vi "Score and Rank Target Objects.vi"(8 "Annotate":bool, 9 "Score Limit":dbl=70.0, 10 "Particles":T4(array[cluster]), 11 "Image in":T3) -> (0 "Target Info":T2(array[cluster]), 3 "Annotated Image":T3)   [LabVIEW 2013]
doc: "Use the location, size, and other factors to score and rank the objects. Optionally show annotations over the objects."
uses:
  <vilib>/vision/Image Controls.llb/IMAQ Image.ctl
  TargetType.ctl
panel:
  out "Numeric":i32
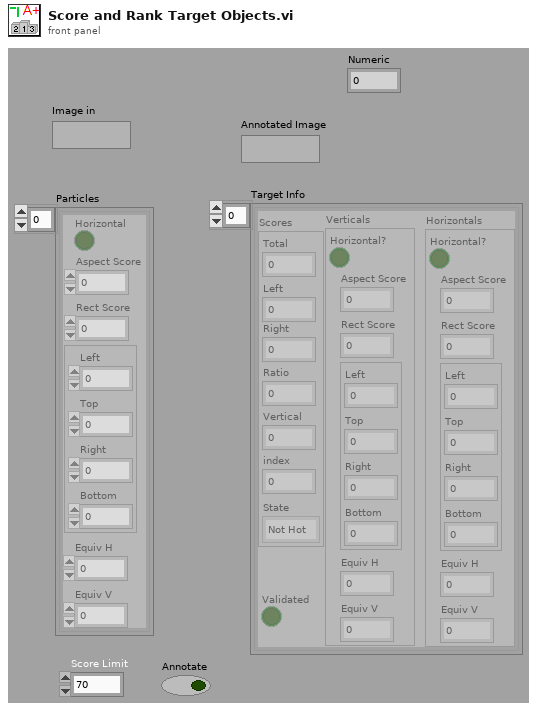
[diagram p1: front panel]
types:
  T1 = typedef "TargetType.ctl" = enum16{"Not Hot", "Hot"}
  T2 = cluster{"Scores":cluster{"Total":dbl, "Left":dbl, "Right":dbl, "Ratio":dbl, "Vertical":dbl, "index":i32, "State":T1}, "Verticals":cluster{"Horizontal?":bool, "Aspect Score":dbl, "Rect Score":dbl, cluster{"Left":dbl, "Top":dbl, "Right":dbl, "Bottom":dbl}, "Equiv H":dbl, "Equiv V":dbl}, "Horizontals":cluster{"Horizontal?":bool, "Aspect Score":dbl, "Rect Score":dbl, cluster{"Left":dbl, "Top":dbl, "Right":dbl, "Bottom":dbl}, "Equiv H":dbl, "Equiv V":dbl}, "Validated":bool}[]
  T3 = typedef "IMAQ Image.ctl" = refnum<image>
  T4 = cluster{"Horizontal":bool, "Aspect Score":dbl, "Rect Score":dbl, cluster{"Left":dbl, "Top":dbl, "Right":dbl, "Bottom":dbl}, "Equiv H":dbl, "Equiv V":dbl}[]
  T5 = cluster{cluster{dbl, dbl, dbl, dbl, dbl, i32, T1}, cluster{"Horizontal":bool, "Aspect Score":dbl, "Rect Score":dbl, cluster{"Left":dbl, "Top":dbl, "Right":dbl, "Bottom":dbl}, "Equiv H":dbl, "Equiv V":dbl}, cluster{"Horizontal":bool, "Aspect Score":dbl, "Rect Score":dbl, cluster{"Left":dbl, "Top":dbl, "Right":dbl, "Bottom":dbl}, "Equiv H":dbl, "Equiv V":dbl}, bool}[]
  T6 = cluster{"Score":dbl, cluster{"Horizontal":bool, "Aspect Score":dbl, "Rect Score":dbl, cluster{"Left":dbl, "Top":dbl, "Right":dbl, "Bottom":dbl}, "Equiv H":dbl, "Equiv V":dbl}}[]
  T7 = cluster{"Horizontal":bool, "Aspect Score":dbl, "Rect Score":dbl, cluster{"Left":dbl, "Top":dbl, "Right":dbl, "Bottom":dbl}, "Equiv H":dbl, "Equiv V":dbl}
  T8 = cluster{cluster{dbl, dbl, dbl, dbl, dbl, i32, T1}, cluster{"Horizontal":bool, "Aspect Score":dbl, "Rect Score":dbl, cluster{"Left":dbl, "Top":dbl, "Right":dbl, "Bottom":dbl}, "Equiv H":dbl, "Equiv V":dbl}, cluster{"Horizontal":bool, "Aspect Score":dbl, "Rect Score":dbl, cluster{"Left":dbl, "Top":dbl, "Right":dbl, "Bottom":dbl}, "Equiv H":dbl, "Equiv V":dbl}, bool}
  T9 = cluster{"Score":dbl, cluster{"Horizontal":bool, "Aspect Score":dbl, "Rect Score":dbl, cluster{"Left":dbl, "Top":dbl, "Right":dbl, "Bottom":dbl}, "Equiv H":dbl, "Equiv V":dbl}}
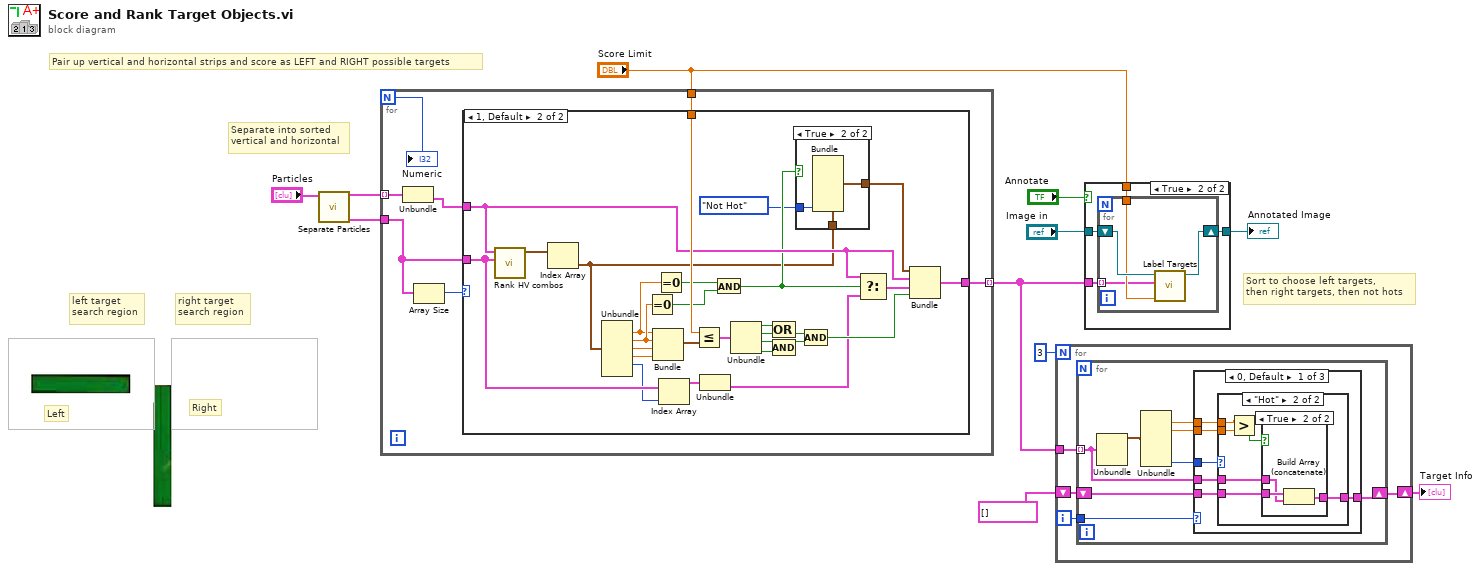
[diagram p0: block diagram]
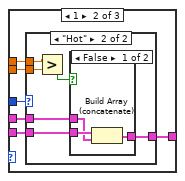
[diagram p5: hidden frame]
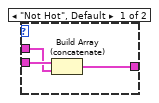
[diagram p9: hidden frame]
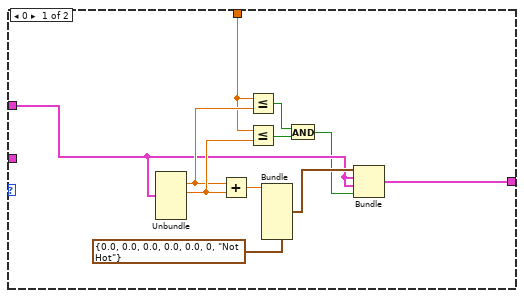
[diagram p10: hidden frame]
diagram:
  # "Sort to choose left targets,\nthen right targets, then not hots"
  # "Right"
  # "Left"
  # "right target\nsearch region"
  # "left target\nsearch region"
  # "Separate into sorted\nvertical and horizontal"
  # "Pair up vertical and horizontal strips and score as LEFT and RIGHT possible targets"
  n1 = call "Separate Particles.vi"("Objects"="Particles") -> ("H Scores"=w7:T6, "V Scores"=w8:T6)  [unwired: 9 in]
  n2 = for {
    N -> [w12]
    tunnel: w8 -> [w18] mode=indexing
    tunnel: w7 -> [w16]
    tunnel: [w14] -> w5 mode=indexing
    tunnel: "Score Limit" -> [w13]
    n3 = Unbundle(w18) -> (w17:T7)  [unwired: 1 out]
    n4 = Array Size(array=w16) -> (size(s)=w15:i32)
    n5 = case shown="1, Default" w15 {
      tunnel: w16 -> [_ w44]
      tunnel: w17 -> [w23 w34]
      tunnel: [w21 w42] -> w14
      tunnel: w13 -> [w20 w41]
      frame 0 {
        n6 = Unbundle(w23) -> ("Aspect Score"=w26:dbl, "Rect Score"=w27:dbl)  [unwired: 4 out]
        n7 = Add(x=w26, y=w27) -> (x+y=w25:dbl)
        n8 = Less Or Equal?(x=w20, y=w26) -> (x <= y?=w28:bool)
        n9 = Less Or Equal?(x=w20, y=w27) -> (x <= y?=w29:bool)
        n10 = Bundle(cluster=cluster{dbl, dbl, dbl, dbl, dbl, i32, T1} {0.0, 0.0, 0.0, 0.0, 0.0, 0, enum."Not Hot"}, w25) -> (w24:cluster{dbl, dbl, dbl, dbl, dbl, i32, T1})  [unwired: 6 in]
        n11 = And(x=w28, y=w29) -> (x .and. y?=w22:bool)
        n12 = Bundle(w24, w23, w23, w22) -> (w21:T8)  [unwired: 1 in]
      }
      frame 1, Default {
        n13 = call "Rank HV combos.vi"("H Scores"=w44, "Vertical"=w34) -> ("Target Scores"=w57:cluster{dbl, dbl, dbl, dbl, dbl, i32, T1}[])  [unwired: 9 in]
        n14 = Index Array(array=w57) -> (element=w30:cluster{dbl, dbl, dbl, dbl, dbl, i32, T1})  [unwired: 1 in]
        n15 = Unbundle(w30) -> (w39:dbl, w40:dbl, w53:dbl, w54:dbl, w43:i32)  [unwired: 2 out]
        n16 = Equal To 0?(x=w40) -> (x = 0?=w37:bool)
        n17 = Bundle(w39, w40, w53, w54) -> (w45:cluster{dbl, dbl, dbl, dbl})  [unwired: 1 in]
        n18 = Equal To 0?(x=w39) -> (x = 0?=w38:bool)
        n19 = Index Array(array=w44, index=w43) -> (element=w55:T9)
        n20 = Less Or Equal?(x=w41, y=w45) -> (x <= y?=w52:cluster{bool, bool, bool, bool})
        n21 = Unbundle(w55) -> (w35:T7)  [unwired: 1 out]
        n22 = And(x=w38, y=w37) -> (x .and. y?=w33:bool)
        n23 = Unbundle(w52) -> (w51:bool, w50:bool, w49:bool, w48:bool)
        n24 = Compound Arithmetic op=OR(w51, w50) -> (w46:bool)
        n25 = Compound Arithmetic op=AND(w49, w48) -> (w47:bool)
        n26 = case shown="True" w33 {
          tunnel: w30 -> [w58 w61]
          tunnel: TargetType."Not Hot" -> [_ w60]
          tunnel: [w58 w59] -> w31
          frame False {
          }
          frame True {
            n27 = Bundle(cluster=w61, w60) -> (w59:cluster{dbl, dbl, dbl, dbl, dbl, i32, T1})  [unwired: 6 in]
          }
        }
        n28 = Compound Arithmetic op=AND(w46, w47) -> (w56:bool)
        n29 = Select(t=w34, s=w33, f=w35) -> (s? t:f=w36:T7)
        n30 = Bundle(w31, w34, w36, w56) -> (w42:T8)  [unwired: 1 in]
      }
    }
    "Numeric" <- w12
  }
  n31 = for {
    N: 3 -> [_]
    tunnel: w5 -> [w65]
    shift-right: [w62] -> w3
    shift-left: T5 [] -> [w63]
    i -> [w64]
    n32 = for {
      tunnel: w65 -> [w69] mode=indexing
      tunnel: w64 -> [w68]
      shift-right: [w66] -> w62
      shift-left: w63 -> [w67]
      n33 = Unbundle(w69) -> (w73:cluster{dbl, dbl, dbl, dbl, dbl, i32, T1})  [unwired: 3 out]
      n34 = Unbundle(w73) -> (w72:dbl, w71:dbl, w70:T1)  [unwired: 4 out]
      n35 = case shown="0, Default" w68 {
        tunnel: w72 -> [w79 w93 w113]
        tunnel: w71 -> [w78 w92 w112]
        tunnel: w70 -> [w75 w91 w111]
        tunnel: w69 -> [w74 w96 w110]
        tunnel: w67 -> [w77 w95 w109]
        tunnel: [w76 w94 w108] -> w66
        frame 0, Default {
          n36 = case shown="\"Hot\"" w75 {
            tunnel: w77 -> [w80 w84]
            tunnel: [w80 w82] -> w76
            tunnel: w79 -> [_ w86]
            tunnel: w78 -> [_ w85]
            tunnel: w74 -> [_ w81]
            frame "Not Hot", Default {
            }
            frame "Hot" {
              n37 = Greater?(x=w86, y=w85) -> (0:w83:bool)
              n38 = case shown="True" w83 {
                tunnel: w84 -> [w87 w90]
                tunnel: [w87 w89] -> w82
                tunnel: w81 -> [_ w88]
                frame False {
                }
                frame True {
                  n39 = Build Array (concatenate)(w90, w88) -> (w89:T5)
                }
              }
            }
          }
        }
        frame 1 {
          n40 = case shown="\"Hot\"" w91 {
            tunnel: w95 -> [w97 w101]
            tunnel: [w97 w99] -> w94
            tunnel: w93 -> [_ w103]
            tunnel: w92 -> [_ w102]
            tunnel: w96 -> [_ w98]
            frame "Not Hot", Default {
            }
            frame "Hot" {
              n41 = Greater?(x=w103, y=w102) -> (0:w100:bool)
              n42 = case shown="False" w100 {
                tunnel: w101 -> [w106 w107]
                tunnel: [w105 w107] -> w99
                tunnel: w98 -> [w104 _]
                frame False {
                  n43 = Build Array (concatenate)(w106, w104) -> (w105:T5)
                }
                frame True {
                }
              }
            }
          }
        }
        frame 2 {
          n44 = case shown="\"Hot\"" w111 {
            tunnel: w113 -> [_ _]
            tunnel: w112 -> [_ _]
            tunnel: w110 -> [w115 _]
            tunnel: w109 -> [w116 w117]
            tunnel: [w114 w117] -> w108
            frame "Not Hot", Default {
              n45 = Build Array (concatenate)(w116, w115) -> (w114:T5)
            }
            frame "Hot" {
            }
          }
        }
      }
    }
  }
  "Target Info" <- w3
  n46 = case shown="True" "Annotate" {
    tunnel: "Image in" -> [w118 w122]
    tunnel: [w118 w121] -> w10
    tunnel: "Score Limit" -> [_ w120]
    tunnel: w5 -> [_ w119]
    frame False {
    }
    frame True {
      n47 = for {
        shift-right: [w123] -> w121
        shift-left: w122 -> [w126]
        tunnel: w119 -> [w124] mode=indexing
        tunnel: w120 -> [w125]
        n48 = call "Label Targets.vi"("Score Limit"=w125, "Target Info"=w124, "Image in"=w126) -> ("Image out"=w123:T3)  [unwired: 8 in]
      }
    }
  }
  "Annotated Image" <- w10
